vi "Global 1.vi"() -> ()   [LabVIEW 2019]
panel:
  out "H3":dbl[][](array[numeric])
  out "HD":dbl[][](array[numeric])
  out "w_ 3":dbl[](array[numeric])
  out "v_ 3":dbl[](array[numeric])
  out "u_ 3":dbl[](array[numeric])
  out "w_ 2":dbl[](array[numeric])
  out "v_ 2":dbl[](array[numeric])
  out "u_ 2":dbl[](array[numeric])
  out "w_1":dbl[](array[numeric])
  out "v_1":dbl[](array[numeric])
  out "u_1":dbl[](array[numeric])
  out "F_measured":dbl[](array[numeric])
  out "a_1 (m)":dbl
  out "L6 (m)":dbl
  out "Rm (m)":dbl
  out "Rf (m)":dbl
  out "Ld (m)":dbl
  out "Lp (m)":dbl
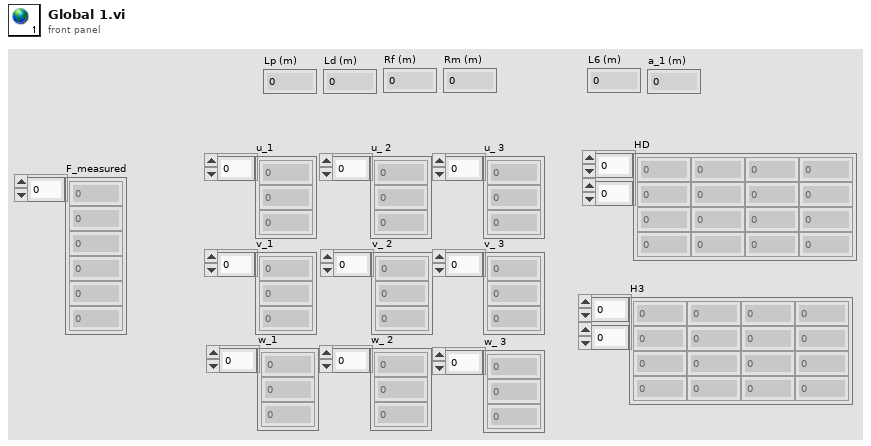
[diagram p1: front panel]
diagram:
